vi "LVClass_WavefrontCorrectorSet Read AllWavefrontCorrectorParametersProperties.vi"(8 "error in (no error)":errorcluster, 11 "WavefrontCorrectorSet in":refnum<class "WavefrontCorrectorSet.lvclass">) -> (0 "error out":errorcluster, 2 "AllWavefrontCorrectorParametersProperties":T1[](array[typedef]), 3 "WavefrontCorrectorSet out":refnum<class "WavefrontCorrectorSet.lvclass">)   [LabVIEW 2020, in "WavefrontCorrectorSet.lvclass"]
uses:
  WavefrontCorrectorSet.lvclass
  Controls/ParameterID.ctl
  Controls/CameraParameters_Type.ctl
  Controls/CameraParameters_Authorization.ctl
  Controls/CameraParameters_OnFlyAuthorization.ctl
  WavefrontCorrectorSet.lvclass/WavefrontCorrectorSet.ctl
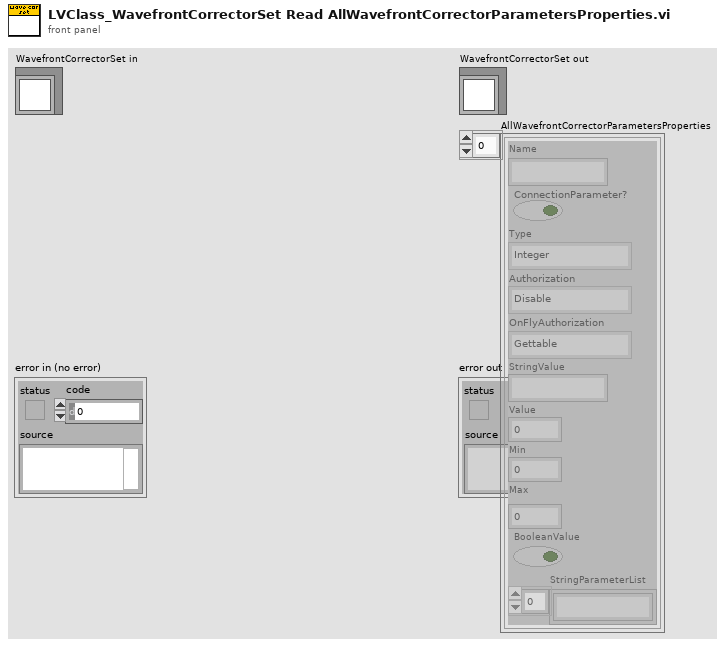
[diagram p1: front panel]
types:
  T1 = typedef "ParameterID.ctl" = cluster{"Name":string, "ConnectionParameter?":bool, "Type":T2, "Authorization":T3, "OnFlyAuthorization":T4, "StringValue":string, "Value":dbl, "Min":dbl, "Max":dbl, "BooleanValue":bool, "StringParameterList":string[]}
  T2 = typedef "CameraParameters_Type.ctl" = enum16{"Integer", "Real", "String", "Boolean"}
  T3 = typedef "CameraParameters_Authorization.ctl" = enum16{"Disable", "Gettable", "Settable - Gettable"}
  T4 = typedef "CameraParameters_OnFlyAuthorization.ctl" = enum16{"None", "Gettable", "Settable", "Settable - Gettable"}
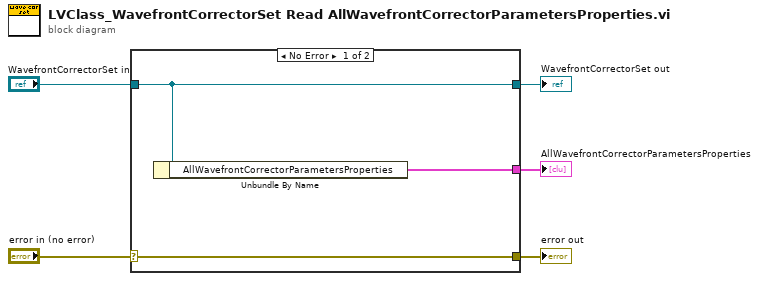
[diagram p0: block diagram]
diagram:
  n1 = case shown="No Error" "error in (no error)" {
    selector: "error in (no error)" -> [w8 w9]
    tunnel: [w8 w9] -> w4
    tunnel: [w7 w10] -> w2
    tunnel: "WavefrontCorrectorSet in" -> [w7 w10]
    tunnel: [w6 _] -> w1
    frame No Error {
      n2 = Unbundle By Name(w7) -> ("AllWavefrontCorrectorParametersProperties"=w6:T1[])
    }
    frame Error {
    }
  }
  "error out" <- w4
  "WavefrontCorrectorSet out" <- w2
  "AllWavefrontCorrectorParametersProperties" <- w1
